vi "GPS Smart.vi"(4 "Factor":cluster{"Kx":dbl, "Ky":dbl, "Kz":dbl}={"Kx"=0.02114, "Ky"=0.0245, "Kz"=0.0705} {"Kz" format="%#_13g"; "Ky" format="%#_13g"; "Kx" format="%#_13g"}, 6 "GPS":cluster{"X":dbl, "Y":dbl, "Angle ":i16}, 8 "Block Rotate":bool, 9 "Set GPS":cluster{"Set":bool, "X":dbl, "Y":dbl, "Z":dbl}, 10 "IMU in":refnum<class "IMU.lvclass">, 11 "Encoders":T1) -> (0 "Ok":bool, 1 "Set GPS Out":cluster{"Set":bool, "X":dbl, "Y":dbl, "Z":dbl}, 3 "GPS True Out":cluster{"X":dbl, "Y":dbl, "Z":dbl})   [LabVIEW 2020]
uses:
  <vilib>/High Genius/HG_WSI_Tookit/Dependencies/Library/IMU/IMU.lvclass
  343eaeb5-5ca9-4ee6-b4f0-e0a9f8e39afa.vi
panel:
  out "IMU":dbl[](array[numeric])
  in  "YAW Old True":dbl
  in  "YAW True":dbl
  in  "GPS True":cluster{"X":dbl, "Y":dbl}
  in  "GPS Old True":cluster{"X":dbl, "Y":dbl}
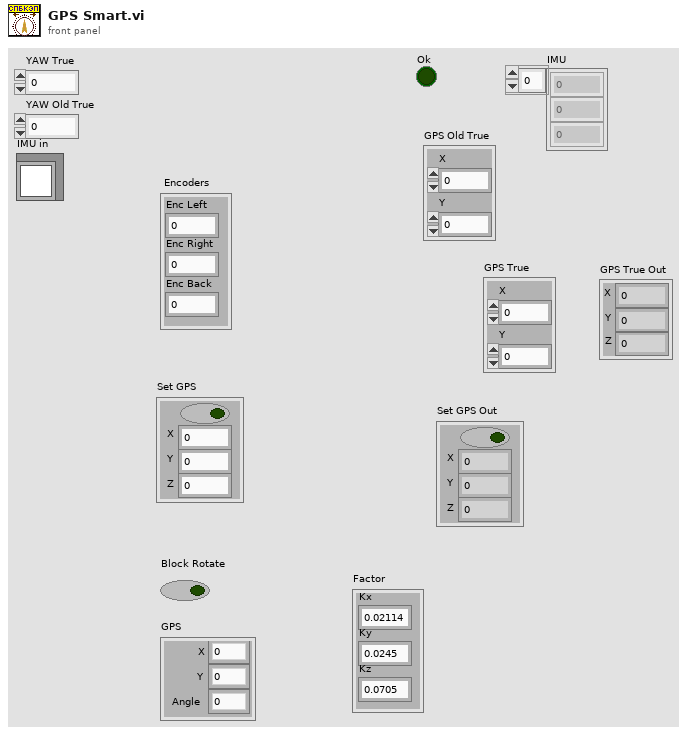
[diagram p1: front panel]
types:
  T1 = cluster{"Enc Left":i32, "Enc Right":i32, "Enc Back":i32}
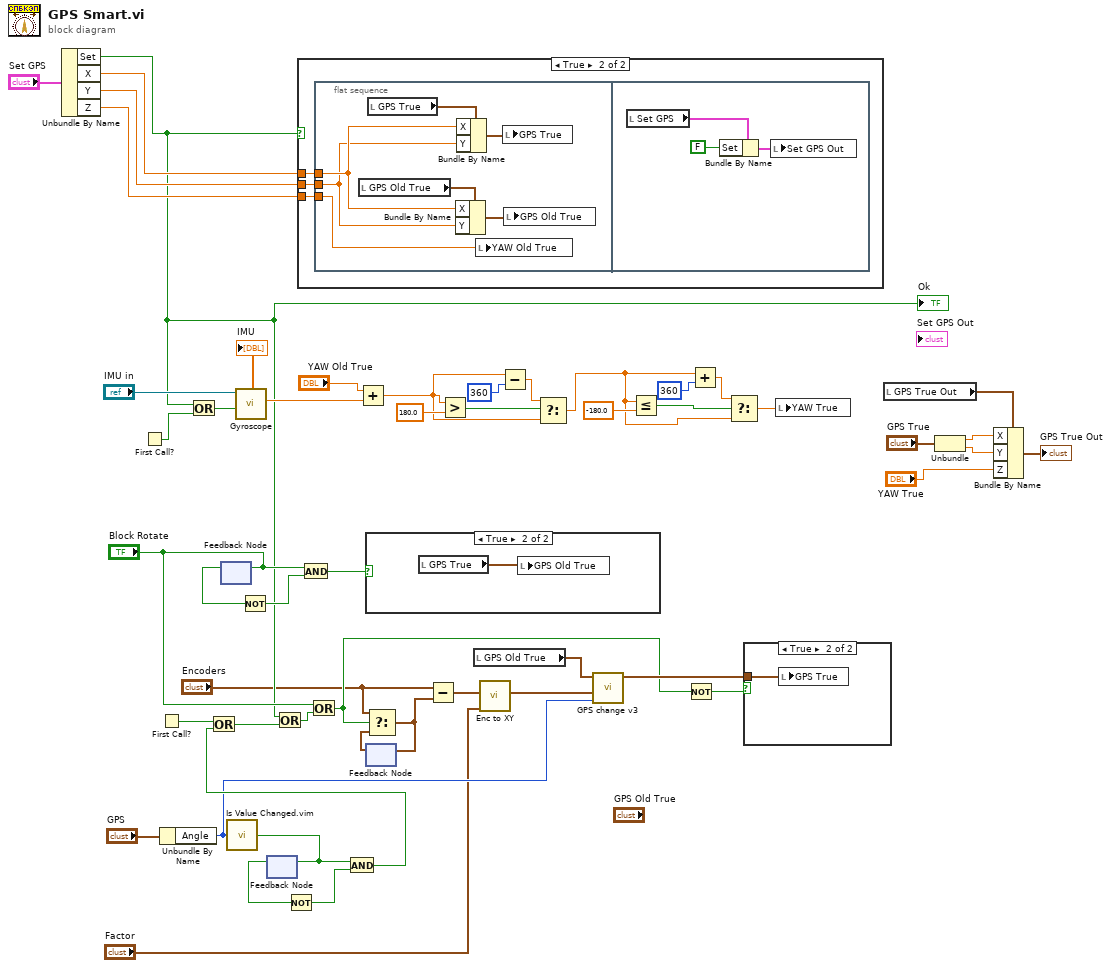
[diagram p0: block diagram]
diagram:
  n1 = Unbundle By Name("Set GPS") -> ("Set"=w16:bool, "X"=w20:dbl, "Y"=w19:dbl, "Z"=w18:dbl)
  "Ok" <- w16
  n2 = First Call?() -> (First Call?: T/F=w22:bool)
  n3 = First Call?() -> (First Call?: T/F=w40:bool)
  n4 = Unbundle By Name("GPS") -> ("Angle"=w34:i16)
  n5 = Or(x=w16, y=w22) -> (x .or. y?=w23:bool)
  n6 = feedback #1() -> (w45:bool)  [unwired: 1 in]
  n7 = feedback-in #1("Block Rotate") -> ()
  n8 = call "Is Value Changed.vim"("value"=w34) -> ("changed or first call?"=w43:bool)
  n9 = call "Gyroscope.vi"("Reset YAW"=w23, "IMU in"="IMU in") -> ("YAW (degree)"=w24:dbl, "IMU"=→"IMU":dbl[])  [unwired: 5 in, 3 out]
  n10 = Not(x=w45) -> (.not. x?=w46:bool)
  n11 = feedback-in #2(w43) -> ()
  n12 = feedback #2() -> (w49:bool)  [unwired: 1 in]
  n13 = Not(x=w49) -> (.not. x?=w48:bool)
  n14 = case shown="True" w16 {
    tunnel: w20 -> [_ w54]
    tunnel: w19 -> [_ w53]
    tunnel: w18 -> [_ w52]
    frame False {
    }
    frame True {
      n15 = flat-sequence {
        tunnel: w54 -> [w59]
        tunnel: w53 -> [w56]
        tunnel: w52 -> [w55]
        frame #0 {
          n16 = local read "GPS Old True"() -> (w58:cluster{"X":dbl, "Y":dbl})
          n17 = local read "GPS True"() -> (w61:cluster{"X":dbl, "Y":dbl})
          n18 = Bundle By Name(cluster=w58, "X"=w59, "Y"=w56) -> (w57:cluster{"X":dbl, "Y":dbl})
          n19 = Bundle By Name(cluster=w61, "X"=w59, "Y"=w56) -> (w60:cluster{"X":dbl, "Y":dbl})
          n20 = local write "YAW Old True"(w55) -> ()
          n21 = local write "GPS True"(w60) -> ()
          n22 = local write "GPS Old True"(w57) -> ()
        }
        frame #1 {
          n23 = local read "Set GPS"() -> (w63:cluster{"Set":bool, "X":dbl, "Y":dbl, "Z":dbl})
          n24 = Bundle By Name(cluster=w63, "Set"=FALSE ("Set X")) -> (w64:cluster{"Set":bool, "X":dbl, "Y":dbl, "Z":dbl})
          n25 = local write "Set GPS Out"(w64) -> ()
        }
      }
    }
  }
  n26 = And(x="Block Rotate", y=w46) -> (x .and. y?=w44:bool)
  n27 = And(x=w43, y=w48) -> (x .and. y?=w39:bool)
  n28 = Or(x=w40, y=w39) -> (x .or. y?=w15:bool)
  n29 = Or(x=w16, y=w15) -> (x .or. y?=w17:bool)
  n30 = Or(x="Block Rotate", y=w17) -> (x .or. y?=w30:bool)
  n31 = Add(x="YAW Old True", y=w24) -> (x+y=w2:dbl)
  n32 = case shown="True" w44 {
    frame False {
    }
    frame True {
      n33 = local read "GPS True"() -> (w65:cluster{"X":dbl, "Y":dbl})
      n34 = local write "GPS Old True"(w65) -> ()
    }
  }
  n35 = feedback #3() -> (w41:T1)  [unwired: 1 in]
  n36 = Select(t="Encoders", s=w30, f=w41) -> (s? t:f=w42:T1)
  n37 = feedback-in #3(w42) -> ()
  n38 = Subtract(x="Encoders", y=w42) -> (x-y=w47:T1)
  n39 = Greater?(x=w2, y=180.0) -> (0:w9:bool)
  n40 = local read "GPS Old True"() -> (w50:cluster{"X":dbl, "Y":dbl})
  n41 = call "Enc to XY.vi"("Factor"="Factor", "Encoders"=w47) -> ("Distance"=w13:cluster{"X":dbl, "Y":dbl})  [unwired: 8 in, 1 out]
  n42 = Subtract(x=w2, y=i16 360) -> (x-y=w8:dbl)
  n43 = Select(t=w8, s=w9, f=w2) -> (s? t:f=w3:dbl)
  n44 = call "GPS change v3.vi"("Angle"=w34, "Change"=w13, "GPS in"=w50) -> ("GPS out"=w33:cluster{"X":dbl, "Y":dbl})  [unwired: 8 in]
  n45 = Less Or Equal?(x=w3, y=-180.0) -> (x <= y?=w7:bool)
  n46 = Not(x=w30) -> (.not. x?=w32:bool)
  n47 = Add(x=w3, y=i16 360) -> (x+y=w5:dbl)
  n48 = Select(t=w5, s=w7, f=w3) -> (s? t:f=w1:dbl)
  n49 = case shown="True" w32 {
    tunnel: w33 -> [_ w66]
    frame False {
    }
    frame True {
      n50 = local write "GPS True"(w66) -> ()
    }
  }
  n51 = local write "YAW True"(w1) -> ()
  n52 = local read "GPS True Out"() -> (w26:cluster{"X":dbl, "Y":dbl, "Z":dbl})
  n53 = Unbundle("GPS True") -> ("X"=w36:dbl, "Y"=w35:dbl)
  n54 = Bundle By Name(cluster=w26, "X"=w36, "Y"=w35, "Z"="YAW True") -> (→"GPS True Out":cluster{"X":dbl, "Y":dbl, "Z":dbl})
